vi "Wait For N Elements Available.vi"(8 "Error in":errorcluster, 9 "N Elements":u32=1, 10 "Timeout (ns)":i64, 11 "CIPC Reference":u64) -> (0 "Error out":errorcluster, 1 "Time Out":bool, 2 "Time Remaining (ns)":i64)   [LabVIEW 2021, in "CIF_NI_CIPC.lvlib"]
doc: "Wait until the N elements, starting from the current reading location, are written by the CIPC writer."
uses:
  CIF_NI_CIPC.lvlib
  <vilib>/Utility/error.llb/Trim Whitespace.vi
  <vilib>/Utility/error.llb/Error Cluster From Error Code.vi
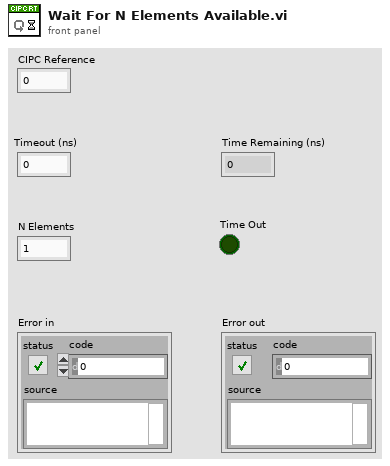
[diagram p1: front panel]
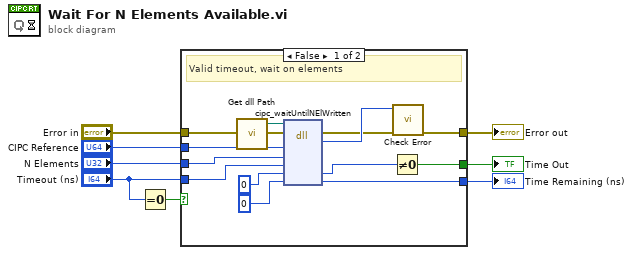
[diagram p0: block diagram]
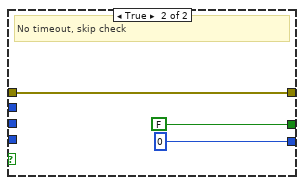
[diagram p2: hidden frame]
diagram:
  n1 = Equal To 0?(x="Timeout (ns)") -> (x = 0?=w1:bool)
  n2 = case shown="False" w1 {
    tunnel: [w19 w24] -> w8
    tunnel: "Timeout (ns)" -> [w18 _]
    tunnel: [w16 i64 0 ("time_left")] -> w7
    tunnel: [w13 FALSE] -> w6
    tunnel: "Error in" -> [w12 w24]
    tunnel: "N Elements" -> [w11 _]
    tunnel: "CIPC Reference" -> [w10 _]
    frame False {
      # "Valid timeout, wait on elements"
      n3 = call "Get dll Path.vi"() -> ("appended path"=w9:path)  [unwired: 5 in]
      n4 = dll-call lib="libnicipc.*" fn="cipc_waitUntilNElWritten"(path in=w9, error in=w12, "cipc_buffer_ref"=w10, "N"=w11, "timeout_ns"=w18, "timed_out"=u8 0 ("timeout_ns"), "time_left"=i64 0 ("timeout_ns")) -> (error out=w20:errorcluster, "return type"=w21:i32, "timed_out"=w14:u8, "time_left"=w16:i64)  [unwired: 4 in, 1 out]
      n5 = Not Equal To 0?(x=w14) -> (x != 0?=w13:bool)
      n6 = call "Check Error.vi"("error in (no error)"=w20, "Error Code"=w21) -> ("error out"=w19:errorcluster)  [unwired: 9 in]
    }
    frame True {
      # "No timeout, skip check"
    }
  }
  "Error out" <- w8
  "Time Out" <- w6
  "Time Remaining (ns)" <- w7
